vi "line2.vi"() -> ()   [LabVIEW 2015]
uses:
  <vilib>/NXT/Block Support/NXT_InputPort.ctl
  <vilib>/NXT/Block Support/NXT_OutputPort.ctl
  <vilib>/NXT/Dual Mode Library/Sensors/Light_On.vi
  <vilib>/NXT/NXTIO Xnodes/NXTIONodeSubVIs/NXTMoveMotors.vi
  <vilib>/NXT/Subs/LVHSConnector.ctl
  <vilib>/NXT/NXTIO Xnodes/AddressXNode/NXTIOAddress.xnode
  <vilib>/NXT/NXTIO Xnodes/NXTIOXNode/NXTIO.xnode
  <vilib>/NXT/LegoClasses/BrickReference/BrickReference.lvclass
  <vilib>/NXT/NXTIO Xnodes/NXTIONodeSubVIs/NXTStopMotors.vi
  <vilib>/NXT/Dual Mode Library/Waits/Wait_Darkness.vi
panel:
  in  "Power/Speed 3":i8=75
  in  "Power/Speed 2":i8=75
  in  "Port (Port 1)":T1=2 items=["Port 1", "Port 2", "Port 3", "Port 4"]
  in  "Power/Speed 1":i8=75
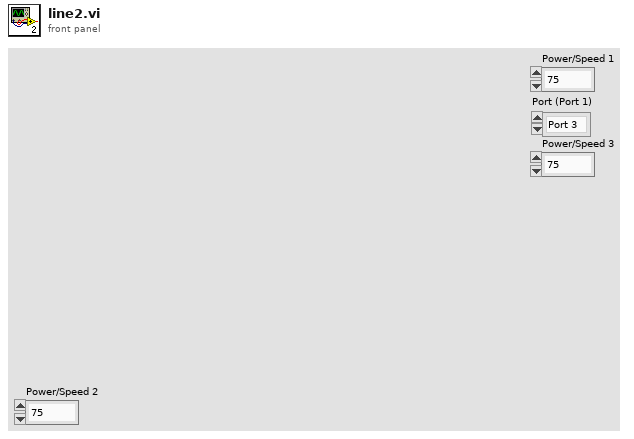
[diagram p1: front panel]
types:
  T1 = typedef "NXT_InputPort.ctl" = u32
  T2 = typedef "NXT_OutputPort.ctl" = u8
  T3 = typedef "LVHSConnector.ctl" = refnum<class "BrickReference.lvclass">
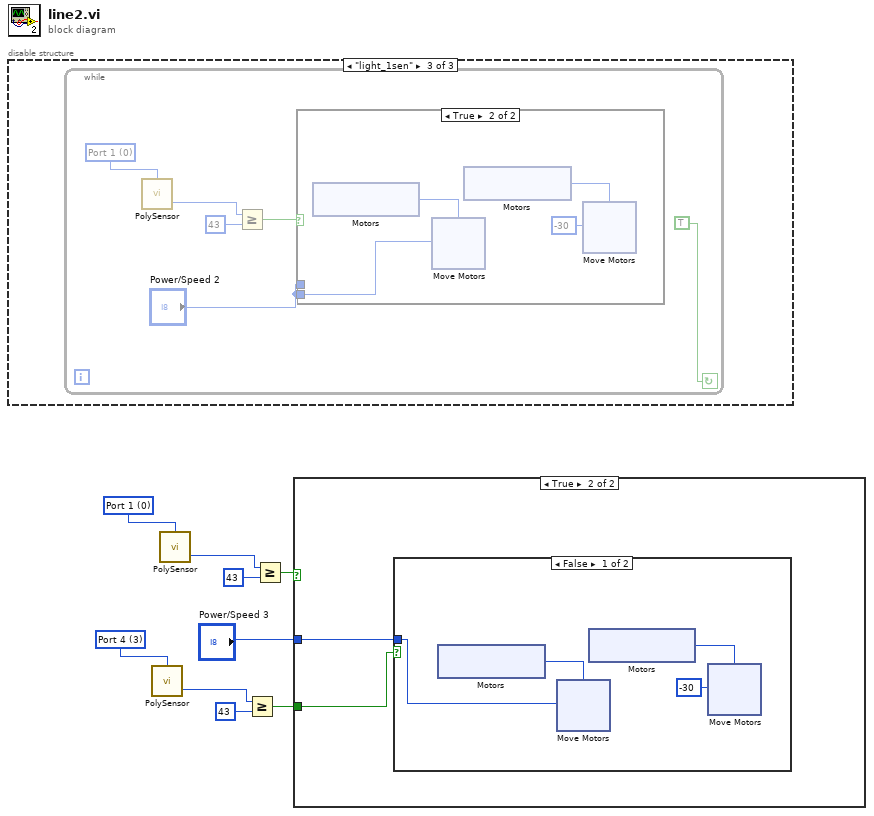
[diagram p0: block diagram]
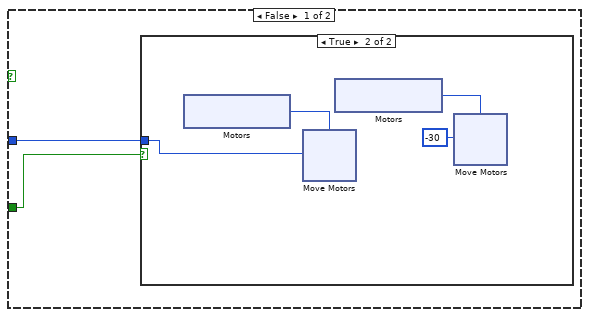
[diagram p2: hidden frame]
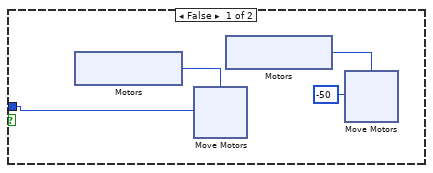
[diagram p3: hidden frame]
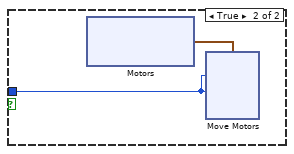
[diagram p4: hidden frame]
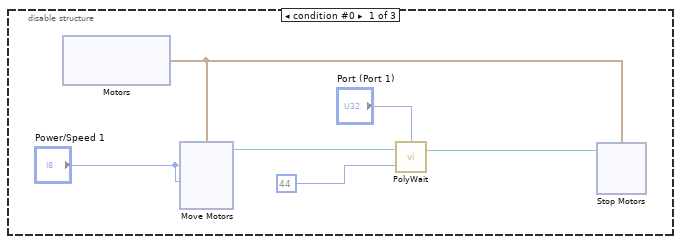
[diagram p5: hidden frame]
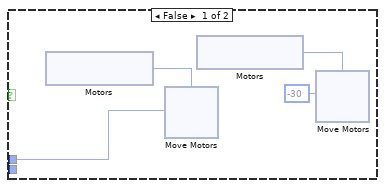
[diagram p7: hidden frame]
diagram:
  w3 = T1 3 items=["Port 1", "Port 2", "Port 3", "Port 4"] ("Port (Port 3)")
  w7 = T1 0 items=["Port 1", "Port 2", "Port 3", "Port 4"] ("Port (Port 3)")
  n1 = disable-structure shown="\"light_1sen\"" {
    frame condition #0 {
      n2 = xnode "Motors"() -> ("Motor"=w15:cluster{"Port":T2, "Port":T2})
      n3 = xnode "Move Motors"("Power/Speed 2"="Power/Speed 1", "Power/Speed 1"="Power/Speed 1", "Motors"=w15) -> ("NXT/EV3"=w13:T3)  [unwired: 1 in]
      n4 = call-poly <vilib>:"PolyWait.vi"("Darkness (40)"=i16 44, "NXT/EV3"=w13, "Port (Port 3)"="Port (Port 1)") -> ("NXT/EV3"=w14:T3)  [unwired: 1 in]
      n5 = xnode "Stop Motors"("Motors"=w15, "NXT/EV3"=w14) -> ()  [unwired: 1 out]
    }
    frame condition #1 (active) {
    }
    frame condition #2 {
      n6 = while {
        stop <- TRUE continue-if-true
        w32 = T1 0 items=["Port 1", "Port 2", "Port 3", "Port 4"] ("Port (Port 3)")
        n7 = call-poly <vilib>:"PolySensor.vi"("Port (Port 3)"=w32) -> ("Scaled Value"=w34:i16)  [unwired: 2 in, 1 out]
        n8 = Greater Or Equal?(x=w34, y=i16 43) -> (x >= y?=w33:bool)
        n9 = case shown="True" w33 {
          tunnel: "Power/Speed 2" -> [_ w59]
          tunnel: "Power/Speed 2" -> [w36 _]
          frame False {
            n10 = xnode "Motors"() -> ("Motor"=w37:T2)
            n11 = xnode "Move Motors"("Power/Speed 1"=w36, "Motors"=w37) -> ()  [unwired: 1 in, 1 out]
            n12 = xnode "Motors"() -> ("Motor"=w38:T2)
            n13 = xnode "Move Motors"("Power/Speed 1"=i8 -30, "Motors"=w38) -> ()  [unwired: 1 in, 1 out]
          }
          frame True {
            n14 = xnode "Motors"() -> ("Motor"=w56:T2)
            n15 = xnode "Move Motors"("Power/Speed 1"=w59, "Motors"=w56) -> ()  [unwired: 1 in, 1 out]
            n16 = xnode "Motors"() -> ("Motor"=w57:T2)
            n17 = xnode "Move Motors"("Power/Speed 1"=i8 -30, "Motors"=w57) -> ()  [unwired: 1 in, 1 out]
          }
        }
      }
    }
  }
  n18 = call-poly <vilib>:"PolySensor.vi"("Port (Port 3)"=w3) -> ("Scaled Value"=w4:i16)  [unwired: 2 in, 1 out]
  n19 = call-poly <vilib>:"PolySensor.vi"("Port (Port 3)"=w7) -> ("Scaled Value"=w8:i16)  [unwired: 2 in, 1 out]
  n20 = Greater Or Equal?(x=w4, y=i16 43) -> (x >= y?=w2:bool)
  n21 = Greater Or Equal?(x=w8, y=i16 43) -> (x >= y?=w6:bool)
  n22 = case shown="True" w6 {
    tunnel: w2 -> [w77 w119]
    tunnel: "Power/Speed 3" -> [w76 w118]
    frame False {
      n23 = case shown="True" w77 {
        tunnel: w76 -> [w78 w98]
        frame False {
          n24 = xnode "Motors"() -> ("Motor"=w79:T2)
          n25 = xnode "Move Motors"("Power/Speed 1"=w78, "Motors"=w79) -> ()  [unwired: 1 in, 1 out]
          n26 = xnode "Motors"() -> ("Motor"=w80:T2)
          n27 = xnode "Move Motors"("Power/Speed 1"=i8 -50, "Motors"=w80) -> ()  [unwired: 1 in, 1 out]
        }
        frame True {
          n28 = xnode "Motors"() -> ("Motor"=w99:T2)
          n29 = xnode "Move Motors"("Power/Speed 1"=w98, "Motors"=w99) -> ()  [unwired: 1 in, 1 out]
          n30 = xnode "Motors"() -> ("Motor"=w100:T2)
          n31 = xnode "Move Motors"("Power/Speed 1"=i8 -30, "Motors"=w100) -> ()  [unwired: 1 in, 1 out]
        }
      }
    }
    frame True {
      n32 = case shown="False" w119 {
        tunnel: w118 -> [w120 w140]
        frame False {
          n33 = xnode "Motors"() -> ("Motor"=w121:T2)
          n34 = xnode "Move Motors"("Power/Speed 1"=w120, "Motors"=w121) -> ()  [unwired: 1 in, 1 out]
          n35 = xnode "Motors"() -> ("Motor"=w122:T2)
          n36 = xnode "Move Motors"("Power/Speed 1"=i8 -30, "Motors"=w122) -> ()  [unwired: 1 in, 1 out]
        }
        frame True {
          n37 = xnode "Motors"() -> ("Motor"=w141:cluster{"Port":T2, "Port":T2})
          n38 = xnode "Move Motors"("Power/Speed 2"=w140, "Power/Speed 1"=w140, "Motors"=w141) -> ()  [unwired: 1 in, 1 out]
        }
      }
    }
  }
